vi "Log_data.vi"(8 "error in (no error)":errorcluster, 11 "Data In":T1) -> (0 "error out":errorcluster)   [LabVIEW 2014]
uses:
  TypeDef/Q1 Message.ctl
  <vilib>/Platform/TimedLoop/XDataNode/timing_clust.ctl
  <vilib>/Platform/TimedLoop/XDataNode/nitl_modes.ctl
  <vilib>/Platform/TimedLoop/XDataNode/wakeup.ctl
  <vilib>/platform/TimedLoop/XDataNode/XDataNode.xnode
  <vilib>/Platform/TimedLoop/XDataNode/XDNodeRunTimeDep.lvlib
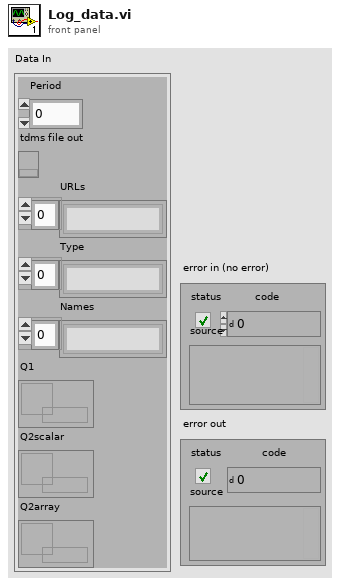
[diagram p1: front panel]
types:
  T1 = cluster{"Period":i64, "tdms file out":refnum<k34>, "URLs":string[], "Type":string[], "Names":string[], "Q1":refnum<queue>, "Q2scalar":refnum<queue>, "Q2array":refnum<queue>}
  T2 = typedef "XDNodeRunTimeDep.lvlib/timing_clust.ctl" = cluster{"Expected End [f-1]":u64, "Actual End [f-1]":u64, "Finished Late? [f-1]":bool, "Expected End [i-1]":u64, "Actual End [i-1]":u64, "Finished Late? [i-1]":bool, "Expected Start [i]":u64, "Actual Start [i]":u64, "Expected Start [f]":u64, "Actual Start [f]":u64, "Source Name":string, "Structure Name":string, "Period":i64, "Deadline":i64, "Offset":i64, "Start":i64, "Priority":i32, "Timeout":i32, "Mode":T3, "Wakeup Reason":T4, "Error":errorcluster, "Source Type":string, "Secondary Source Type":string, "Global End Time":u64, "Global Start Time":u64, "Frame Duration":u64, "Iteration Duration":u64, "Assigned CPU":i32, "I/O Scan Engine Mode":u32}
  T3 = typedef "XDNodeRunTimeDep.lvlib/nitl_modes.ctl" = enum32{"No Change", "Process missed periods, maintain original phase", "Discard missed periods, maintain original phase", "Process missed periods, ignore original phase", "Discard missed periods, ignore original phase"}
  T4 = typedef "XDNodeRunTimeDep.lvlib/wakeup.ctl" = enum32{"Normal", "Aborted", "Asynchronous wakeup", "Timing source error", "Timed loop error", "Timeout"}
  T5 = typedef "Q1 Message.ctl" = cluster{"state":enum16{"initialize", "idle", "preparation", "record", "stop", "exit", "defrag", "View"}, "data":variant}
  T6 = enum16{"initialize", "idle", "preparation", "record", "stop", "exit", "defrag", "View"}
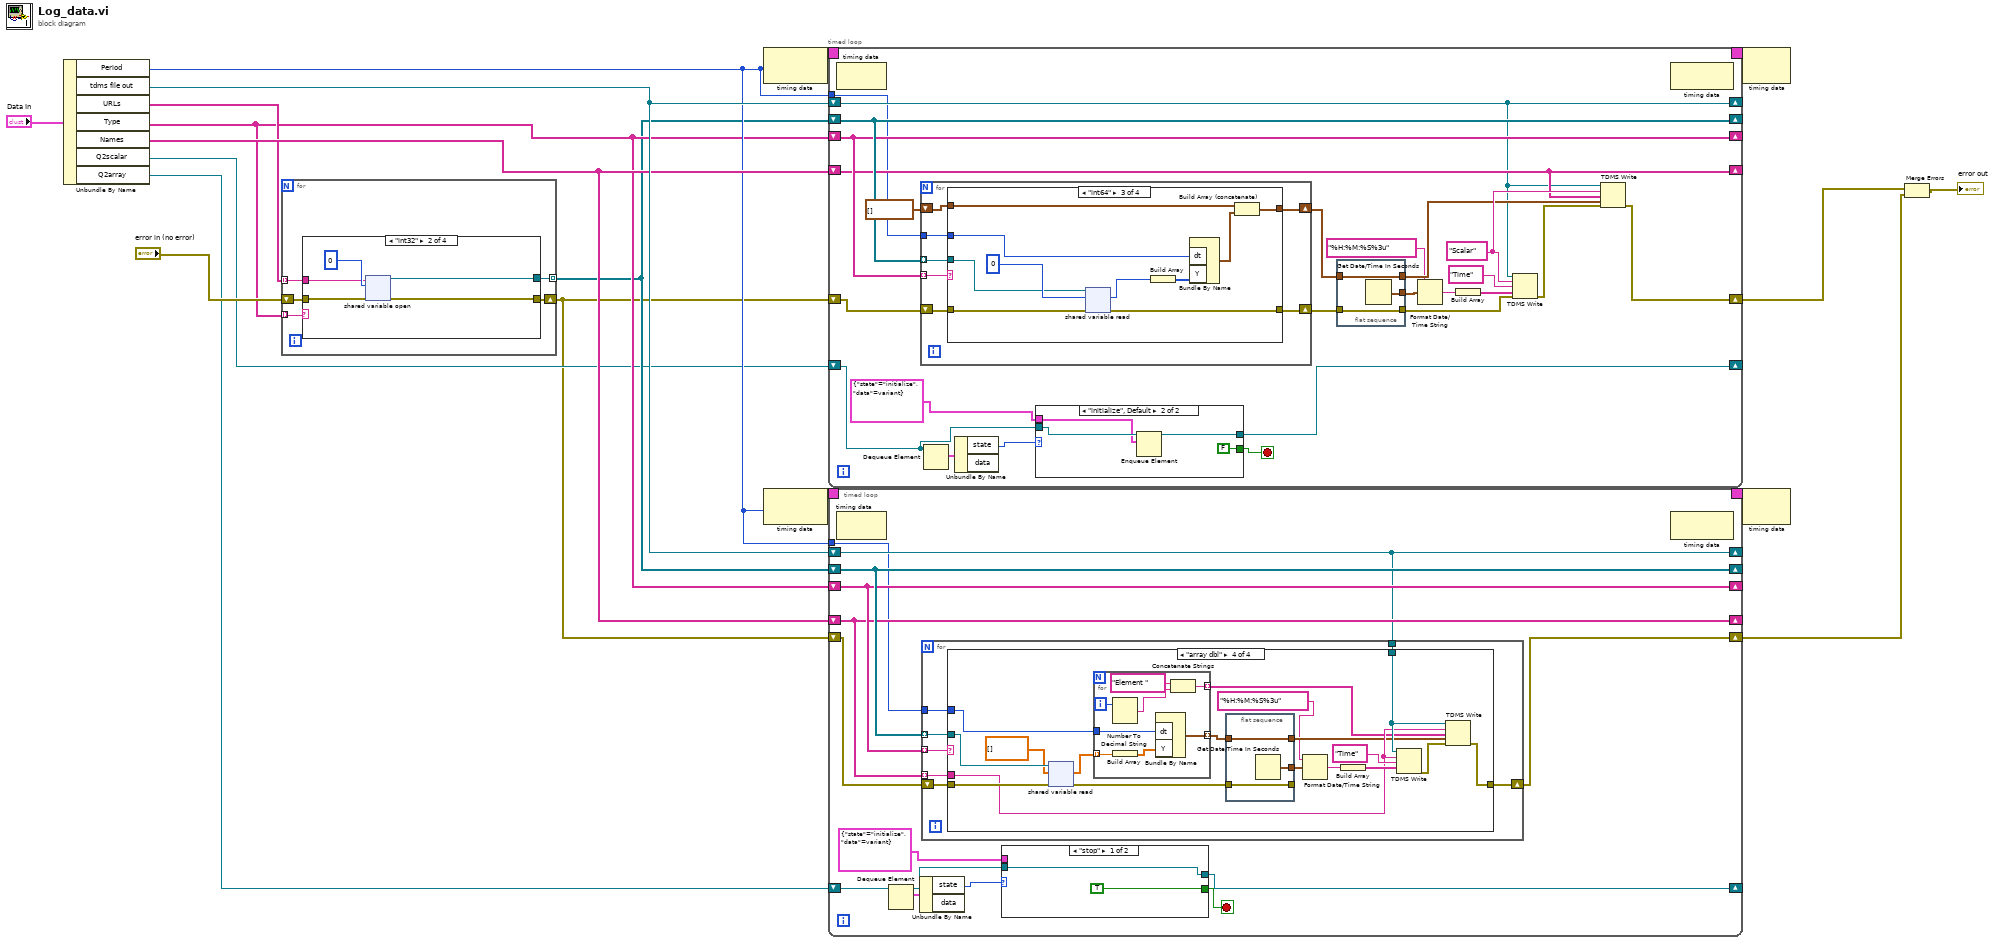
[diagram p0: block diagram]
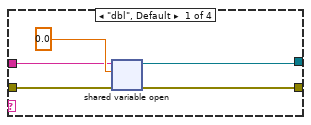
[diagram p2: hidden frame]
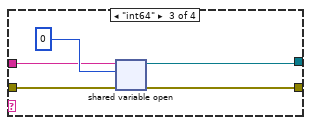
[diagram p3: hidden frame]
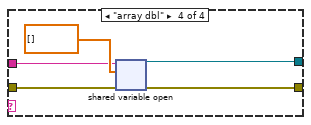
[diagram p4: hidden frame]
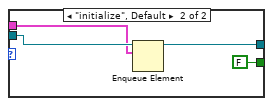
[diagram p5: hidden frame]
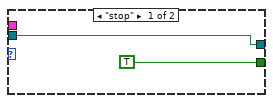
[diagram p9: hidden frame]
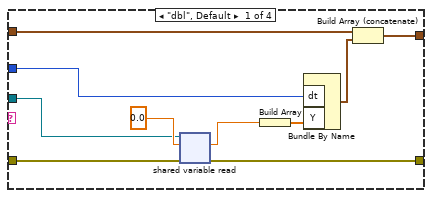
[diagram p10: hidden frame]
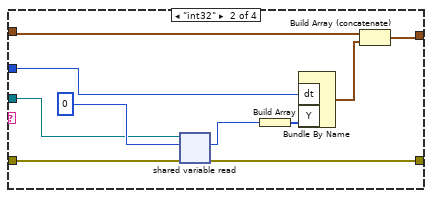
[diagram p11: hidden frame]
diagram:
  n1 = Unbundle By Name("Data In") -> ("Period"=w11:i64, "tdms file out"=w13:refnum<k34>, "URLs"=w9:string[], "Type"=w8:string[], "Names"=w12:string[], "Q2scalar"=w3:refnum<queue>, "Q2array"=w2:refnum<queue>)
  n2 = for {
    shift-right: [w21] -> w1
    shift-left: "error in (no error)" -> [w23]
    tunnel: [w22] -> w7 mode=indexing
    tunnel: w9 -> [w20] mode=indexing
    tunnel: w8 -> [w19] mode=indexing
    n3 = case shown="\"int32\"" w19 {
      tunnel: w23 -> [w27 w32 w37 w41]
      tunnel: [w26 w30 w35 w42] -> w22
      tunnel: [w25 w31 w36 w43] -> w21
      tunnel: w20 -> [w24 w29 w34 w39]
      frame "dbl", Default {
        n4 = shared-variable-open(w24, w27, 0.0) -> (w26:refnum<k21>, w25:errorcluster)  [unwired: 1 in]
      }
      frame "int32" {
        n5 = shared-variable-open(w29, w32, 0) -> (w30:refnum<k21>, w31:errorcluster)  [unwired: 1 in]
      }
      frame "int64" {
        n6 = shared-variable-open(w34, w37, i64 0) -> (w35:refnum<k21>, w36:errorcluster)  [unwired: 1 in]
      }
      frame "array dbl" {
        n7 = shared-variable-open(w39, w41, dbl[] []) -> (w42:refnum<k21>, w43:errorcluster)  [unwired: 1 in]
      }
    }
  }
  n8 = node-c288(w11) -> (w18:T2)
  n9 = node-c288(w11) -> (w16:T2)
  n10 = timed-loop {
    timing: w18 -> [_]
    timing-out: [_] -> w17
    shift-right: [w67] -> _
    shift-left: w7 -> [w67]
    shift-right: [w66] -> _
    shift-left: w8 -> [w66]
    shift-right: [w55] -> _
    shift-left: w13 -> [w55]
    shift-right: [w49] -> w6
    shift-left: w1 -> [w68]
    shift-right: [w56] -> _
    shift-left: w12 -> [w56]
    tunnel: w11 -> [w53]
    shift-right: [w46] -> _
    shift-left: w3 -> [w47]
    stop <- w48 stop-if-true
    w58 = "Scalar"
    n11 = node-c288() -> ()  [unwired: 1 in, 1 out]
    n12 = for {
      tunnel: w67 -> [w83] mode=indexing
      tunnel: w66 -> [w84] mode=indexing
      shift-right: [w81] -> w65
      shift-left: w68 -> [w82]
      tunnel: w53 -> [w80]
      shift-right: [w78] -> w64
      shift-left: waveform(dbl)[] [] -> [w79]
      n13 = case shown="\"int64\"" w84 {
        tunnel: w83 -> [w91 w101 w111 _]
        tunnel: w82 -> [w90 w100 w110 w115]
        tunnel: [w89 w99 w109 w115] -> w81
        tunnel: w80 -> [w88 w98 w108 _]
        tunnel: w79 -> [w87 w96 w105 w116]
        tunnel: [w86 w97 w107 w116] -> w78
        frame "dbl", Default {
          n14 = shared-variable-read(w91, w90, 0.0) -> (w89:errorcluster, w92:dbl)  [unwired: 2 out]
          n15 = Build Array(w92) -> (w93:dbl[])
          n16 = Bundle By Name("dt"=w88, "Y"=w93) -> (w85:waveform(dbl))  [unwired: 1 in]
          n17 = Build Array (concatenate)(w87, w85) -> (w86:waveform(dbl)[])
        }
        frame "int32" {
          n18 = shared-variable-read(w101, w100, 0) -> (w99:errorcluster, w102:i32)  [unwired: 2 out]
          n19 = Build Array(w102) -> (w103:i32[])
          n20 = Bundle By Name("dt"=w98, "Y"=w103) -> (w95:waveform(i32))  [unwired: 1 in]
          n21 = Build Array (concatenate)(w96, w95) -> (w97:waveform(dbl)[])
        }
        frame "int64" {
          n22 = shared-variable-read(w111, w110, i64 0) -> (w109:errorcluster, w112:i64)  [unwired: 2 out]
          n23 = Build Array(w112) -> (w113:i64[])
          n24 = Bundle By Name("dt"=w108, "Y"=w113) -> (w106:waveform(i64))  [unwired: 1 in]
          n25 = Build Array (concatenate)(w105, w106) -> (w107:waveform(dbl)[])
        }
        frame "array dbl" {
        }
      }
    }
    n26 = Dequeue Element(queue=w47) -> (element=w51:T5)  [unwired: 2 in, 3 out]
    n27 = Unbundle By Name(w51) -> ("state"=w50:T6)  [unwired: 1 out]
    n28 = case shown="\"initialize\", Default" w50 {
      tunnel: [TRUE FALSE] -> w48
      tunnel: w47 -> [w69 w73]
      tunnel: T5 {"state"=enum."initialize", "data"=variant} ("Q1 Message") -> [_ w72]
      tunnel: [w69 w71] -> w46
      frame "stop" {
      }
      frame "initialize", Default {
        n29 = Enqueue Element(queue=w73, element=w72) -> (queue out=w71:refnum<queue>)  [unwired: 2 in, 2 out]
      }
    }
    n30 = flat-sequence {
      tunnel: w65 -> [w76]
      tunnel: w64 -> [w75]
      tunnel: [w77] -> w63
      tunnel: [w76] -> w59
      tunnel: [w75] -> w57
      frame #0 {
        n31 = Get Date/Time In Seconds() -> (seconds since 1Jan1904=w77:timestamp)
      }
    }
    n32 = Format Date/Time String(time format string (%c)="%H:%M:%S%3u", seconds (now)=w63) -> (date/time string=w62:string)  [unwired: 1 in]
    n33 = Build Array(w62) -> (w61:string[])
    n34 = TDMS Write(0:w55, 5:w58, 7:"Time", 9:w61, 11:w59) -> (15:w52:errorcluster)  [unwired: 1 in, 3 out]
    n35 = TDMS Write(0:w55, 5:w58, 7:w56, 9:w57, 11:w52) -> (15:w49:errorcluster)  [unwired: 1 in, 3 out]
    n36 = node-c288() -> ()  [unwired: 1 in, 1 out]
  }
  n37 = timed-loop {
    timing: w16 -> [_]
    timing-out: [_] -> w15
    shift-right: [w131] -> _
    shift-left: w7 -> [w131]
    shift-right: [w130] -> _
    shift-left: w8 -> [w130]
    shift-right: [w128] -> _
    shift-left: w13 -> [w128]
    shift-right: [w120] -> w5
    shift-left: w1 -> [w132]
    shift-right: [w129] -> _
    shift-left: w12 -> [w129]
    tunnel: w11 -> [w127]
    shift-right: [w121] -> _
    shift-left: w2 -> [w126]
    stop <- w119 stop-if-true
    n38 = node-c288() -> ()  [unwired: 1 in, 1 out]
    n39 = Dequeue Element(queue=w126) -> (queue out=w123:refnum<queue>, element=w125:T5)  [unwired: 2 in, 2 out]
    n40 = Unbundle By Name(w125) -> ("state"=w124:T6)  [unwired: 1 out]
    n41 = for {
      tunnel: w131 -> [w144] mode=indexing
      tunnel: w130 -> [w145] mode=indexing
      shift-right: [w142] -> w120
      shift-left: w132 -> [w143]
      tunnel: w127 -> [w141]
      tunnel: w129 -> [w140] mode=indexing
      tunnel: w128 -> [w139]
      n42 = case shown="\"array dbl\"" w145 {
        tunnel: w144 -> [_ _ _ w165]
        tunnel: w143 -> [w146 w147 w148 w164]
        tunnel: [w146 w147 w148 w150] -> w142
        tunnel: w141 -> [_ _ _ w163]
        tunnel: w140 -> [_ _ _ w154]
        tunnel: w139 -> [_ _ _ w155]
        frame "dbl", Default {
        }
        frame "int32" {
        }
        frame "int64" {
        }
        frame "array dbl" {
          n43 = shared-variable-read(w165, w164, dbl[] []) -> (w161:errorcluster, w166:dbl[])  [unwired: 2 out]
          n44 = for {
            tunnel: w166 -> [w177] mode=indexing
            tunnel: w163 -> [w176]
            tunnel: [w175] -> w160 mode=indexing
            tunnel: [w170] -> w153 mode=indexing
            i -> [w173]
            n45 = Number To Decimal String(number=w173) -> (decimal integer string=w171:string)  [unwired: 1 in]
            n46 = Build Array(w177) -> (w174:dbl[])
            n47 = Bundle By Name("dt"=w176, "Y"=w174) -> (w175:waveform(dbl))  [unwired: 1 in]
            n48 = Concatenate Strings("Element ", w171) -> (w170:string)
          }
          n49 = flat-sequence {
            tunnel: w161 -> [w169]
            tunnel: w160 -> [w168]
            tunnel: [w169] -> _
            tunnel: [w168] -> w151
            tunnel: [w167] -> w156
            frame #0 {
              n50 = Get Date/Time In Seconds() -> (seconds since 1Jan1904=w167:timestamp)
            }
          }
          n51 = Format Date/Time String(time format string (%c)="%H:%M:%S%3u", seconds (now)=w156) -> (date/time string=w159:string)  [unwired: 1 in]
          n52 = Build Array(w159) -> (w158:string[])
          n53 = TDMS Write(0:w155, 5:w154, 7:"Time", 9:w158) -> (15:w152:errorcluster)  [unwired: 2 in, 3 out]
          n54 = TDMS Write(0:w155, 5:w154, 7:w153, 9:w151, 11:w152) -> (15:w150:errorcluster)  [unwired: 1 in, 3 out]
        }
      }
    }
    n55 = case shown="\"stop\"" w124 {
      tunnel: [TRUE FALSE] -> w119
      tunnel: w123 -> [w133 w137]
      tunnel: T5 {"state"=enum."initialize", "data"=variant} ("Q1 Message") -> [_ w136]
      tunnel: [w133 w135] -> w121
      frame "stop" {
      }
      frame "initialize", Default {
        n56 = Enqueue Element(queue=w137, element=w136) -> (queue out=w135:refnum<queue>)  [unwired: 2 in, 2 out]
      }
    }
    n57 = node-c288() -> ()  [unwired: 1 in, 1 out]
  }
  n58 = node-c288(w17) -> ()  [unwired: 1 out]
  n59 = node-c288(w15) -> ()  [unwired: 1 out]
  n60 = Merge Errors(w6, w5) -> (→"error out":errorcluster)
